vi "Configuration Reference.vi"(8 "Error in":errorcluster, 11 "Sample Test Template in":refnum<class "Sample Test Template.lvclass">) -> (0 "Error out":errorcluster, 2 "VI Ref":refnum<vi>, 3 "Sample Test Template out":refnum<class "Sample Test Template.lvclass">)   [LabVIEW 2020, in "Sample Test Template.lvclass"]
doc: "Dynamic method for configuration page reference"
uses:
  Sample Test Template.lvclass
  Parent/Typedef/LV2 Control.ctl
  Configuration Page.vi
  Parent/Test.lvclass
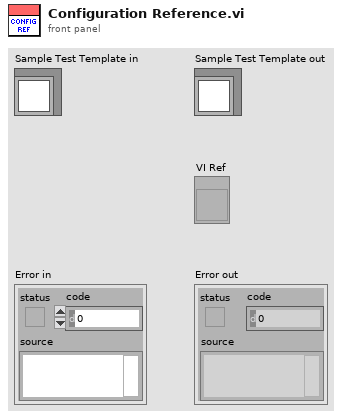
[diagram p1: front panel]
types:
  T1 = typedef "Test.lvclass/LV2 Control.ctl" = enum16{"Home", "Mode", "Config", "Status", "Read"}
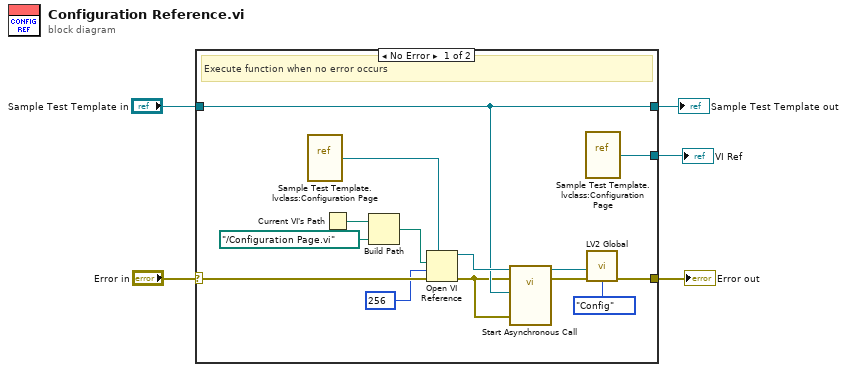
[diagram p0: block diagram]
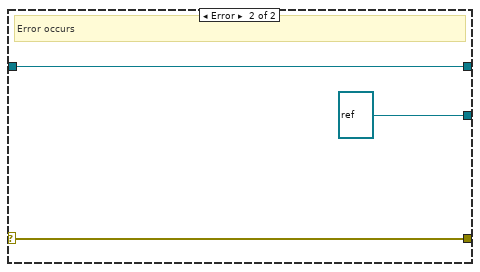
[diagram p2: hidden frame]
diagram:
  n1 = case shown="No Error" "Error in" {
    selector: "Error in" -> [w16 w22]
    tunnel: [w8 w22] -> w2
    tunnel: "Sample Test Template in" -> [w11 w20]
    tunnel: [w19 refnum<vi> refnum] -> w3
    tunnel: [w11 w20] -> w4
    frame No Error {
      # "Execute function when no error occurs"
      n2 = vi-ref "Sample Test Template.lvclass:Configuration Page.vi"() -> (w14:refnum<vi>)
      n3 = Current VI's Path() -> (path=w18:path)
      n4 = Build Path(base path=w18, name or relative path=path "../Configuration Page.vi") -> (appended path=w15:path)
      n5 = Open VI Reference(type specifier VI Refnum (for type only)=w14, vi path=w15, options=256, error in (no error)=w16) -> (vi reference=w12:refnum<vi>, error out=w10:errorcluster)  [unwired: 2 in]
      n6 = call-by-ref "Start Asynchronous Call"(reference=w12, error in=w10, "Error In"=w10, "Sample Test Template in"=w11) -> (reference out=w7:refnum<vi>, error out=w9:errorcluster)  [unwired: 8 in, 2 out]
      n7 = vi-ref "Sample Test Template.lvclass:Configuration Page.vi"() -> (w19:refnum<vi>)
      n8 = call "LV2 Global.vi"("Configuration Ref In"=w7, "Error In"=w9, "Enum"=LV2_Control."Config") -> ("Error Out"=w8:errorcluster)  [unwired: 8 in, 4 out]
    }
    frame Error {
      # "Error occurs"
    }
  }
  "Error out" <- w2
  "Sample Test Template out" <- w4
  "VI Ref" <- w3
